vi "oa_TV Extract Geometric Imperfection (Digital Tacho NChan).vi"(0 "digital tacho info":T1[](array[typedef]), 3 "reset? (F)":bool, 7 "pulse/revolution":i32[](array[numeric]), 11 "error in (no error)":errorcluster) -> (4 "pulse positions":cluster{dbl[]}[](array[cluster]), 8 "revulotion":i32[](array[numeric]), 10 "revulotion index":i32[](array[numeric]), 15 "error out":errorcluster)   [LabVIEW 2017, in "SoundVib_Torsional.lvlib"]
uses:
  <vilib>/addons/Sound and Vibration/Order Analysis/Torsional Vibration/SoundVib_Torsional.lvlib
  <vilib>/addons/Sound and Vibration/Order Analysis/Tach Process/SubVIs/digital tach info.ctl
  <vilib>/addons/Sound and Vibration/Order Analysis/Tach Process/SubVIs/oa_Process Counter Data (N Tach).vi
  <vilib>/addons/Sound and Vibration/Order Analysis/Tach Process/SoundVib_TachProcess.lvlib
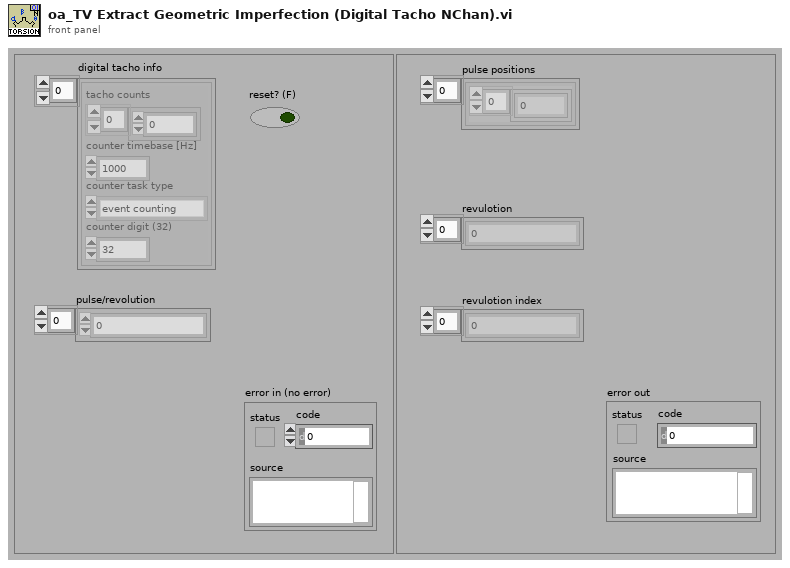
[diagram p1: front panel]
types:
  T1 = typedef "SoundVib_TachProcess.lvlib/digital tach info.ctl" = cluster{"tacho counts":i64[], "counter timebase [Hz]":dbl, "counter task type":enum16{"period measurement", "event counting"}, "counter digit (32)":i32}
  T2 = cluster{"pulse positions [s]":dbl[], "counter timebase [Hz]":dbl, "counter task type":enum16{"period measurement", "event counting"}, "counter digit":i32}[]
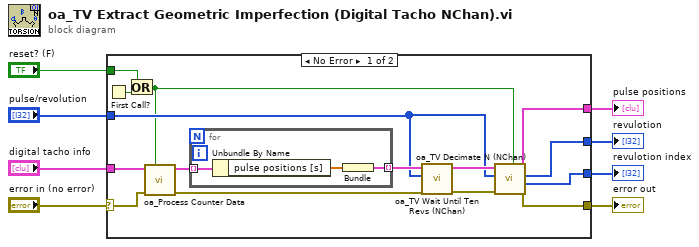
[diagram p0: block diagram]
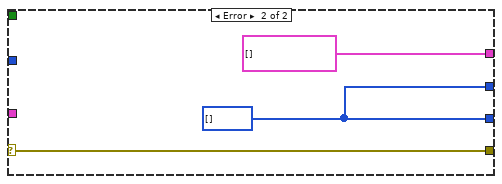
[diagram p2: hidden frame]
diagram:
  n1 = case shown="No Error" "error in (no error)" {
    selector: "error in (no error)" -> [w21 w29]
    tunnel: "pulse/revolution" -> [w16 _]
    tunnel: [w12 w29] -> w7
    tunnel: "digital tacho info" -> [w23 _]
    tunnel: [w14 w28] -> w4
    tunnel: [w13 w28] -> w3
    tunnel: [w11 cluster{dbl[]}[] [] ("angle intervals")] -> w2
    tunnel: "reset? (F)" -> [w9 _]
    frame No Error {
      n2 = First Call?() -> (First Call?: T/F=w10:bool)
      n3 = Or(x=w9, y=w10) -> (x .or. y?=w15:bool)
      n4 = call-poly <vilib>:"oa_Process Counter Data.vi"("reset?(True)"=w15, "error in (no error)"=w21, "digital tach info"=w23) -> ("error out (no error)"=w17:errorcluster, "digital tach info out (DBL)"=w22:T2)  [unwired: 7 in]
      n5 = for {
        tunnel: w22 -> [w26] mode=indexing
        tunnel: [w25] -> w18 mode=indexing
        n6 = Unbundle By Name(w26) -> ("pulse positions [s]"=w24:dbl[])
        n7 = Bundle("pulse positions [s]"=w24) -> (w25:cluster{"pulse positions [s]":dbl[]})  [unwired: 1 in]
      }
      n8 = call <vilib>:"oa_TV Wait Until Ten Revs (NChan).vi"("error in (no error)"=w17, "pulse/revolution"=w16, "pulse position [s]"=w18) -> ("error out"=w19:errorcluster, "pulse positions"=w20:cluster{dbl[]}[])  [unwired: 7 in]
      n9 = call <vilib>:"oa_TV Decimate N (NChan).vi"("reset? (F)"=w15, "error in (no error)"=w19, "pulse/revolution"=w16, "pulse position [s]"=w20) -> ("error out"=w12:errorcluster, "revulotion index"=w13:i32[], "revulotion"=w14:i32[], "pulse positions"=w11:cluster{dbl[]}[])  [unwired: 4 in]
    }
    frame Error {
      w28 = i32[] [] ("revulotion")
    }
  }
  "error out" <- w7
  "revulotion index" <- w3
  "revulotion" <- w4
  "pulse positions" <- w2
